vi "parse_token_test.vi"() -> ()   [LabVIEW 2015]
panel:
  out "ok":bool
  out "response_metadata":cluster{"next_cursor":string}
  out "channel":T1
  out "error out":errorcluster
  out "Cluster":T2
  in  "body":string
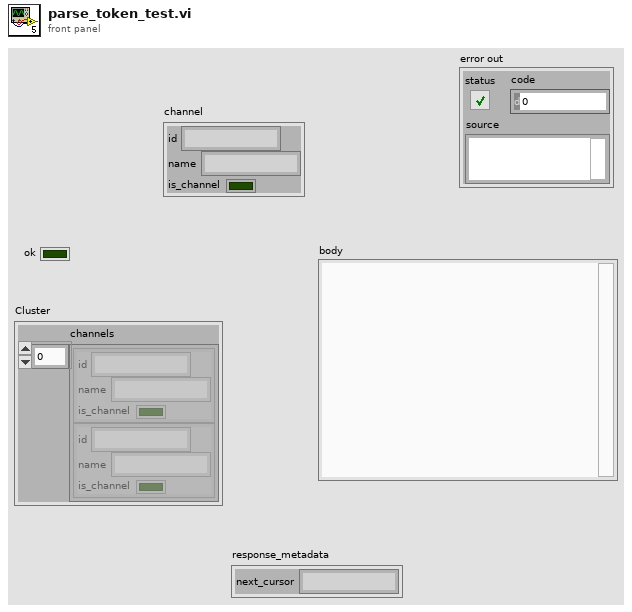
[diagram p1: front panel]
types:
  T1 = cluster{"id":string, "name":string, "is_channel":bool}
  T2 = cluster{"channels":cluster{"id":string, "name":string, "is_channel":bool}[]}
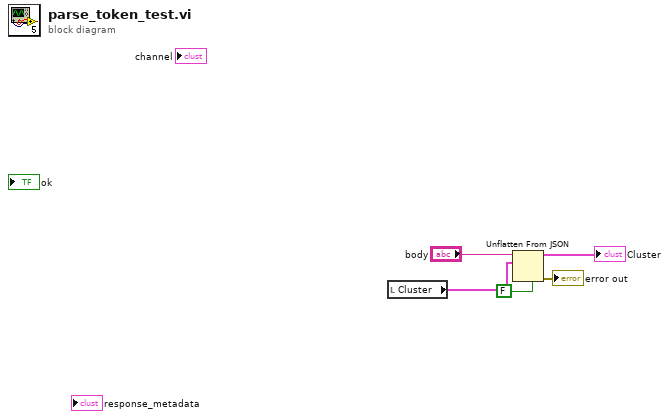
[diagram p0: block diagram]
diagram:
  n1 = local read "Cluster"() -> (w4:T2)
  n2 = Unflatten From JSON(JSON string="body", type and defaults=w4, strict validation? (F)=FALSE) -> (value=→"Cluster":T2, error out=→"error out":errorcluster)  [unwired: 4 in]
